vi "nn reallocmsg.vi"(8 "error in (no error)":errorcluster, 10 "size":u32, 11 "msg":u32) -> (0 "error out":errorcluster, 2 "function return":u32, 3 "msg out":u32)   [LabVIEW 2013, in "lvnano.lvlib"]
doc: "NN_EXPORT void *nn_reallocmsg (void *msg, size_t size);"
uses:
  lvnano.lvlib
  get last error code.vi
  get error string from code.vi
  <vilib>/Utility/error.llb/Error Cluster From Error Code.vi
  lvnanomsg.dll
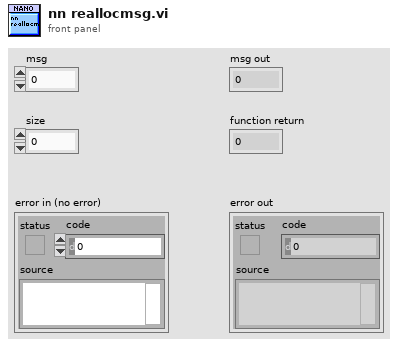
[diagram p1: front panel]
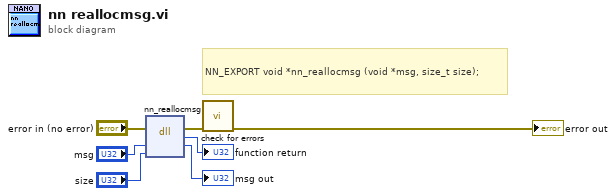
[diagram p0: block diagram]
diagram:
  # "NN_EXPORT void *nn_reallocmsg (void *msg, size_t size);"
  n1 = dll-call lib="C:/Users/Daniel/Documents/nanomsg/lvnano/lvnanomsg.*" fn="nn_reallocmsg"(error in="error in (no error)", "msg"="msg", "size"="size") -> (error out=w2:errorcluster, →"function return":u32, "msg"=→"msg out":u32)  [unwired: 3 in, 1 out]
  n2 = call "check for errors.vi"("error in"=w2) -> ("error out"=→"error out":errorcluster)  [unwired: 10 in]
